vi "removeFirstLineAttributes.vi"(8 "error in (no error)":errorcluster, 10 "XMLString in":string) -> (0 "error out":errorcluster, 2 "XMLString out":string)   [LabVIEW 2014, in "XML.lvlib" / "XMLAttributeParser.lvclass"]
doc: "This method removes first line attributes for methods that cannot handle attributes in the first line."
uses:
  <userlib>/Common/XML/XMLAttributeParser/XMLAttributeParser.lvclass
panel:
  # "<dAz_ArcsPS type=\"cool\">0</dAz_ArcsPS>"
  # "<difftrack class=\"TCSDataDefinitions::TCSCommand:TargetConfiguration.Target.DifftrackAzEl\" version=\"1.5\" type=\"awesome\">\n  <dAz_ArcsPS type=\"cool\">0</dAz_ArcsPS>\n  <dEl_ArcsPS>0</dEl_ArcsPS>\n</difftrack>"
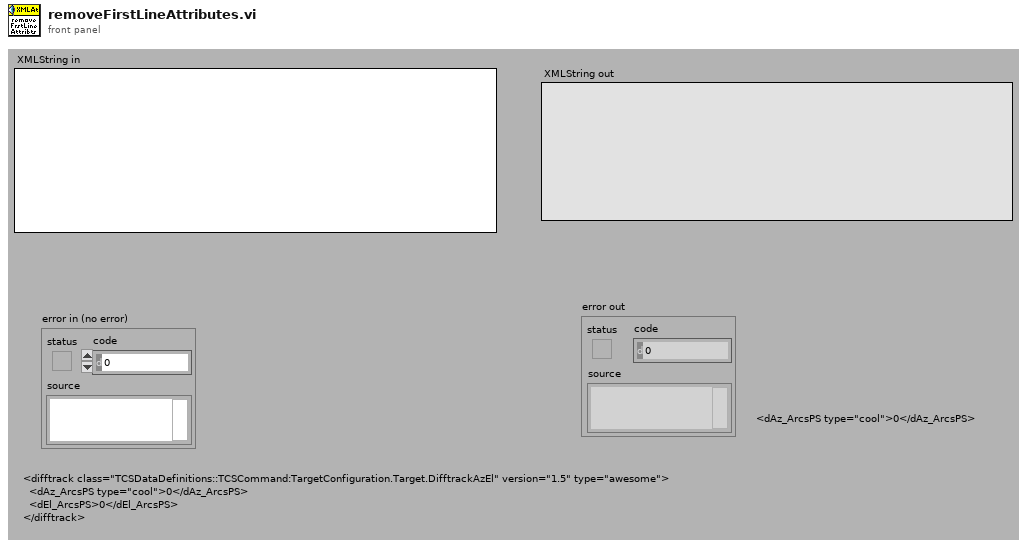
[diagram p1: front panel]
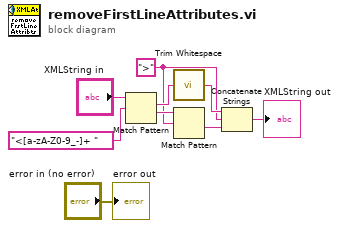
[diagram p0: block diagram]
diagram:
  w3 = ">" ("string")
  n1 = Match Pattern(string="XMLString in", regular expression="<[a-zA-Z0-9_-]+ ") -> (match substring=w6:string, after substring=w4:string)  [unwired: 1 in, 2 out]
  n2 = call <vilib>:"Trim Whitespace.vi"("string"=w6) -> ("trimmed string"=w5:string)  [unwired: 1 in]
  n3 = Match Pattern(string=w4, regular expression=w3) -> (after substring=w2:string)  [unwired: 1 in, 3 out]
  n4 = Concatenate Strings(w5, w3, w2) -> (→"XMLString out":string)
  "error out" <- "error in (no error)"
